vi "RP-ANALOG-OUT.vi"(1 "Voltage":dbl, 2 "Pin #":u16(ring) items=["AOUT0", "AOUT1", "AOUT2", "AOUT3"], 3 "IP address":string="192.168.4.129") -> (0 "error out":errorcluster)   [LabVIEW 2021]
uses:
  Variance measurement/Red_Pitaya/RedPitaya.lvlib
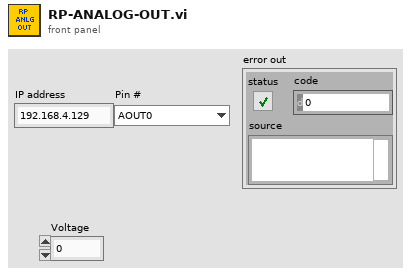
[diagram p1: front panel]
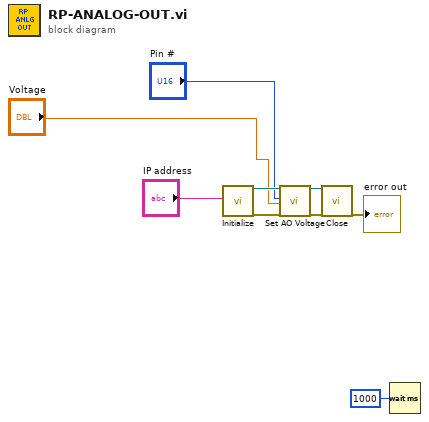
[diagram p0: block diagram]
diagram:
  n1 = call "Initialize.vi"("IP address"="IP address") -> ("RedPitaya connection out"=w9:refnum<k5>, "error out"=w8:errorcluster)  [unwired: 17 in]
  n2 = call "Set AO Voltage.vi"("RedPitaya connection in"=w9, "Pin #"="Pin #", "Analog Voltage Value (V)"="Voltage", "error in"=w8) -> ("RedPitaya connection out"=w6:refnum<k5>, "error out"=w7:errorcluster)  [unwired: 14 in]
  n3 = call "Close.vi"("RedPitaya connection in"=w6, "error in"=w7) -> ("error out"=→"error out":errorcluster)  [unwired: 17 in]
  n4 = Wait (ms)(milliseconds to wait=u32 1000 ("attente (ms)")) -> ()  [unwired: 1 out]
